vi "SwerveAssistHeading.vi"(1 "Joystick X":dbl, 2 "Joystick Y":dbl, 3 "In Deadband":bool, 4 "Joystick Rotation":dbl, 5 "Rotation Maximum":dbl=1.0, 6 "Locked Heading (deg) [0,360]":dbl format="%#_13g", 7 "Heading Angle PID":T1={"Kp"=0.1, "Ki"=0.1, "Kd"=0.1, "N-Diff"=10, "N-Int"=20, "Int Error Window"=0.5, "Max Ouput"=1.0, "Min Output"=-1.0, "Square Derivative"=FALSE, "N-Prop"=1} {"N-Prop" min=1; "Int Error Window" min=0.0; "N-Int" min=2; "N-Diff" min=2; "Kd" min=0.0; "Ki" min=0.0; "Kp" min=0.0}, 9 "Anti-Drift PID":T1={"Kp"=0.1, "Ki"=0.1, "Kd"=0.1, "N-Diff"=10, "N-Int"=20, "Int Error Window"=0.5, "Max Ouput"=1.0, "Min Output"=-1.0, "Square Derivative"=FALSE, "N-Prop"=1} {"N-Prop" min=1; "Int Error Window" min=0.0; "N-Int" min=2; "N-Diff" min=2; "Kd" min=0.0; "Ki" min=0.0; "Kp" min=0.0}, 10 "Orientation Mode":enum16{"Robot-Oriented", "Field-Oriented"}(ring), 11 "Heading Fudge Max (deg)":dbl=10.0, 13 "Deceleration Hysteresis (ms)":u32=250) -> (14 "Heading PID Plot":T2, 17 "In Deadband":bool, 18 "Assisted Rotation":dbl, 19 "Heading Assist On":bool)   [LabVIEW 2020]
doc: "This VI runs PID controllers to maintain the robot's heading using either (1) a locked heading angle or (2) preventing the robot from drifting while translating above a specified velocity. Dropping below the velocity threshold or manually commanding a rotation will switch off the anti-drift heading lock."
uses:
  b65aea0e-782f-4c6a-b3da-6b6dab4b3ae4.vi
  GlobalDrivebase.vi
  GlobalPoseAndTargeting.vi
  GlobalDriverStationData.vi
  GlobalDriverStationCommands.vi
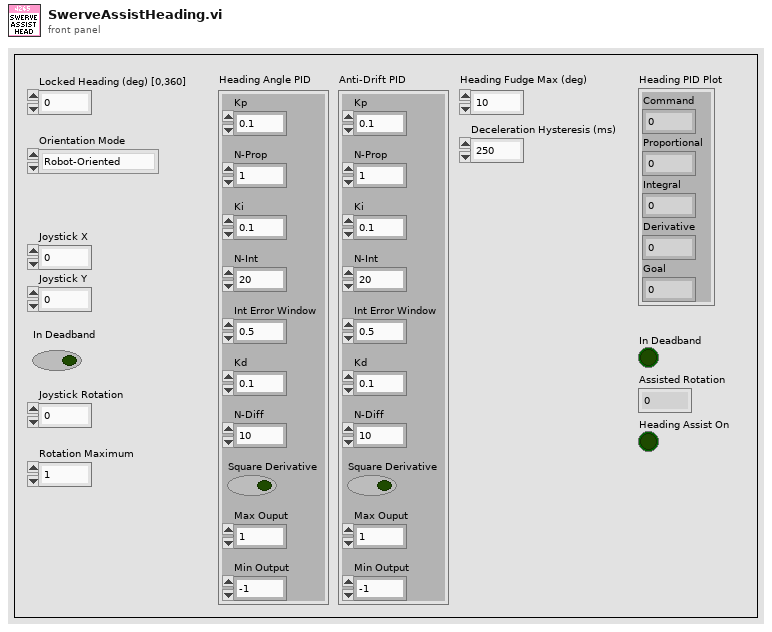
[diagram p1: front panel]
types:
  T1 = cluster{"Kp":dbl, "Ki":dbl, "Kd":dbl, "N-Diff":i32, "N-Int":i32, "Int Error Window":dbl, "Max Ouput":dbl, "Min Output":dbl, "Square Derivative":bool, "N-Prop":i32}
  T2 = cluster{"Command":dbl, "Proportional":dbl, "Integral":dbl, "Derivative":dbl, "Goal":dbl}
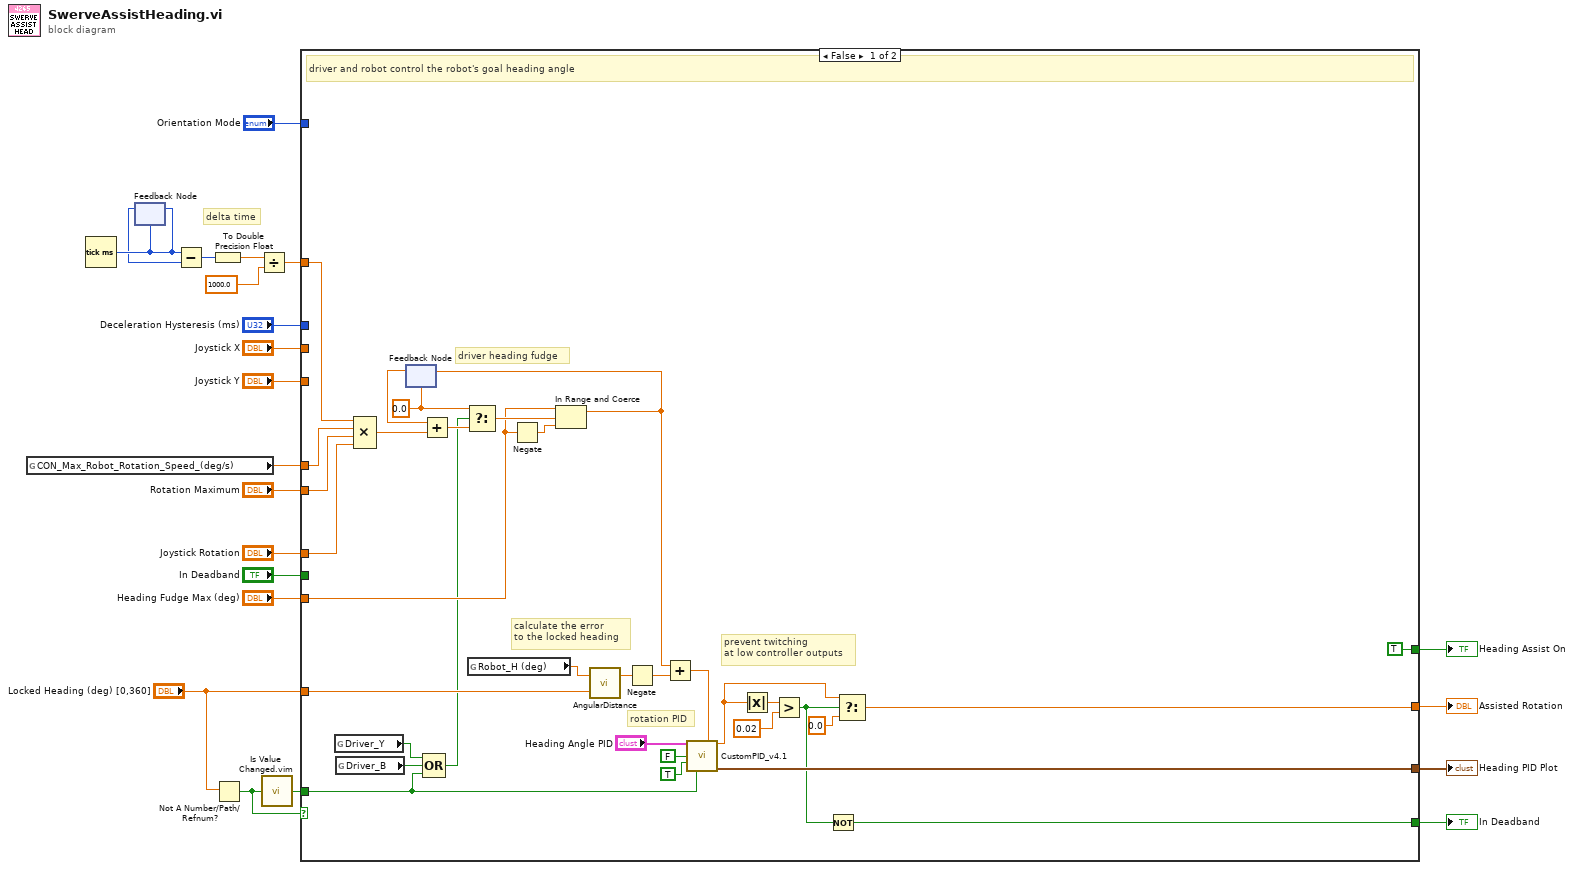
[diagram p0: block diagram]
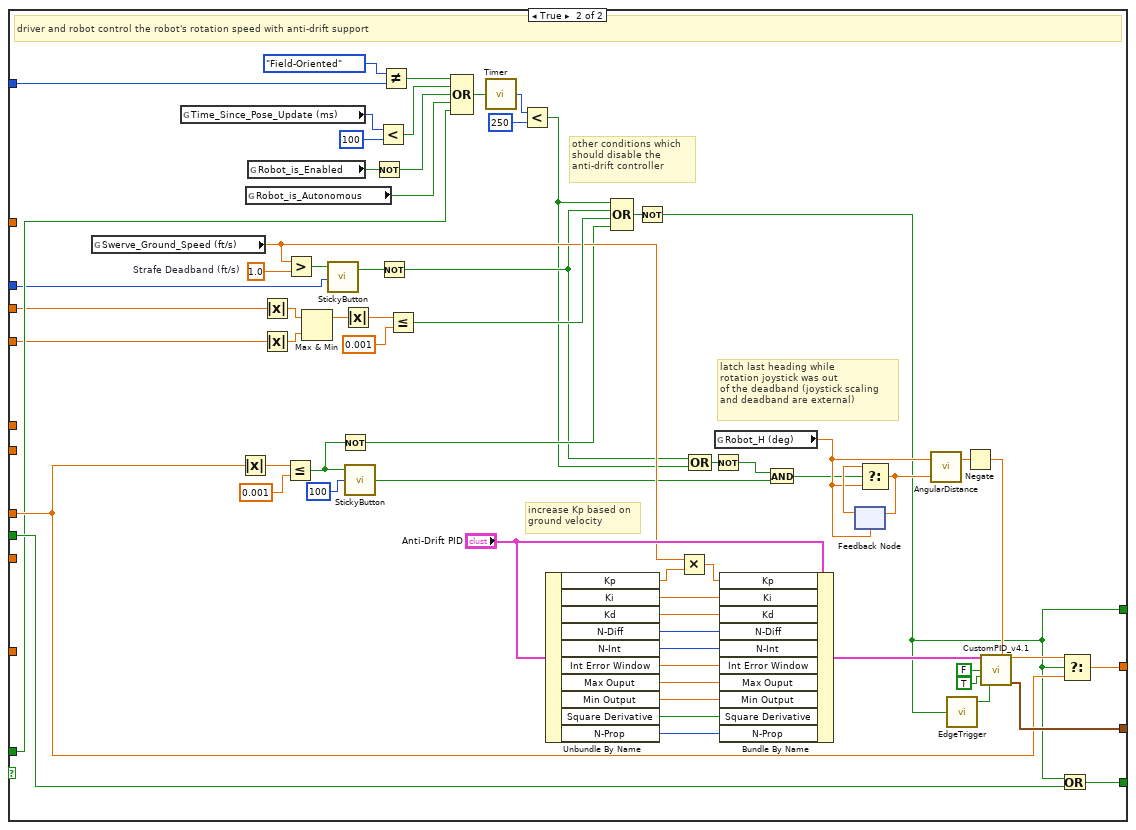
[diagram p2: hidden frame]
diagram:
  # "delta time"
  n1 = global read "GlobalDrivebase.vi" "CON_Max_Robot_Rotation_Speed_(deg/s)"() -> (w17:dbl)
  n2 = Tick Count (ms)() -> (millisecond timer value=w16:u32)
  n3 = feedback #1(w16) -> (w15:u32)
  n4 = feedback-in #1(w16) -> ()
  n5 = Subtract(x=w16, y=w15) -> (x-y=w14:u32)
  n6 = To Double Precision Float(number=w14) -> (double precision float=w13:dbl)
  n7 = Not A Number/Path/Refnum?(number/path/refnum="Locked Heading (deg) [0,360]") -> (NaN/Path/Refnum?=w20:bool)
  n8 = Divide(x=w13, y=1000.0) -> (x/y=w11:dbl)
  n9 = call "Is Value Changed.vim"("value"=w20) -> ("changed or first call?"=w5:bool)
  n10 = case shown="False" w20 {
    tunnel: "Locked Heading (deg) [0,360]" -> [w48 _]
    tunnel: [w47 w83] -> w8
    tunnel: "Joystick Rotation" -> [w38 w81]
    tunnel: [w42 w82] -> w9
    tunnel: [w28 w80] -> w7
    tunnel: w5 -> [w25 w63]
    tunnel: "In Deadband" -> [_ w79]
    tunnel: w17 -> [w40 _]
    tunnel: "Rotation Maximum" -> [w39 _]
    tunnel: w11 -> [w37 _]
    tunnel: "Heading Fudge Max (deg)" -> [w30 _]
    tunnel: [TRUE w78] -> w6
    tunnel: "Deceleration Hysteresis (ms)" -> [_ w62]
    tunnel: "Joystick Y" -> [_ w58]
    tunnel: "Joystick X" -> [_ w57]
    tunnel: "Orientation Mode" -> [_ w56]
    frame False {
      w33 = 0.0
      # "driver heading fudge"
      # "prevent twitching\nat low controller outputs"
      # "rotation PID"
      # "calculate the error\nto the locked heading"
      # "driver and robot control the robot's goal heading angle"
      n11 = global read "GlobalDriverStationCommands.vi" "Driver_Y"() -> (w23:bool)
      n12 = global read "GlobalDriverStationCommands.vi" "Driver_B"() -> (w26:bool)
      n13 = Compound Arithmetic op=MULTIPLY(w37, w40, w39, w38) -> (w36:dbl)
      n14 = feedback #2(w33) -> (w34:dbl)
      n15 = Add(x=w34, y=w36) -> (x+y=w35:dbl)
      n16 = Compound Arithmetic op=OR(w23, w26, w25) -> (w24:bool)
      n17 = Select(t=w33, s=w24, f=w35) -> (s? t:f=w31:dbl)
      n18 = global read "GlobalPoseAndTargeting.vi" "Robot_H (deg)"() -> (w55:dbl)
      n19 = Negate(x=w30) -> (-x=w32:dbl)
      n20 = In Range and Coerce(upper limit=w30, x=w31, lower limit=w32) -> (coerced(x)=w29:dbl)  [unwired: 1 out]
      n21 = feedback-in #2(w29) -> ()
      n22 = call "AngularDistance.vi"("Goal Angle (deg) [0,360]"=w48, "Current Angle (deg) [-Inf,+Inf]"=w55) -> ("Signed Angular Distance (deg) [-180,+180]"=w54:dbl)  [unwired: 1 out]
      n23 = Negate(x=w54) -> (-x=w49:dbl)
      n24 = Add(x=w29, y=w49) -> (x+y=w53:dbl)
      n25 = call "CustomPID_v4.1.vi"("PID Tuning Parameters"="Heading Angle PID", "Custom Error Calculation"=w53, "Reset on Goal Change ?"=FALSE, "Use Custom Error Calculation ?"=TRUE, "Reinit"=w25) -> ("Command"=w44:dbl, "Controller Summary"=w47:T2)  [unwired: 7 in, 2 out]
      n26 = Absolute Value(x=w44) -> (abs(x)=w46:dbl)
      n27 = Greater?(x=w46, y=0.02) -> (0:w41:bool)
      n28 = Not(x=w41) -> (.not. x?=w28:bool)
      n29 = Select(t=w44, s=w41, f=0.0 ("t")) -> (s? t:f=w42:dbl)
    }
    frame True {
      w112 = 1.0  # Strafe Deadband (ft/s)
      # "other conditions which\nshould disable the\nanti-drift controller"
      # "increase Kp based on\nground velocity"
      # "latch last heading while\nrotation joystick was out \nof the deadband (joystick scaling \nand deadband are external)"
      # "driver and robot control the robot's rotation speed with anti-drift support"
      n30 = global read "GlobalPoseAndTargeting.vi" "Swerve_Ground_Speed (ft/s)"() -> (w93:dbl)
      n31 = global read "GlobalPoseAndTargeting.vi" "Time_Since_Pose_Update (ms)"() -> (w70:u32)
      n32 = Absolute Value(x=w81) -> (abs(x)=w117:dbl)
      n33 = global read "GlobalDriverStationData.vi" "Robot_is_Autonomous"() -> (w67:bool)
      n34 = global read "GlobalDriverStationData.vi" "Robot_is_Enabled"() -> (w69:bool)
      n35 = Absolute Value(x=w57) -> (abs(x)=w61:dbl)
      n36 = Absolute Value(x=w58) -> (abs(x)=w60:dbl)
      n37 = Less Or Equal?(x=w117, y=0.001) -> (x <= y?=w85:bool)
      n38 = Greater?(x=w93, y=w112) -> (0:w87:bool)
      n39 = Max & Min(x=w61, y=w60) -> (max(x,y)=w59:dbl)  [unwired: 1 out]
      n40 = call "StickyButton.vi"("Time threshold (ms)"=w62, "Button Input"=w87) -> ("Sticky Button"=w88:bool)  [unwired: 1 in]
      n41 = Not(x=w85) -> (.not. x?=w66:bool)
      n42 = Absolute Value(x=w59) -> (abs(x)=w98:dbl)
      n43 = call "StickyButton.vi"("Time threshold (ms)"=u32 100 ("y"), "Button Input"=w85) -> ("Sticky Button"=w86:bool)  [unwired: 1 in]
      n44 = Not(x=w69) -> (.not. x?=w68:bool)
      n45 = Less?(x=w70, y=u32 100) -> (x < y?=w76:bool)
      n46 = Not(x=w88) -> (.not. x?=w65:bool)
      n47 = Not Equal?(x=enum16{"Robot-Oriented", "Field-Oriented"}."Field-Oriented", y=w56) -> (x != y?=w75:bool)
      n48 = Less Or Equal?(x=w98, y=0.001) -> (x <= y?=w96:bool)
      n49 = Compound Arithmetic op=OR(w75, w76, w68, w67, w63) -> (w73:bool)
      n50 = call "Timer.vi"("Reset Timer"=w73) -> ("Time (ms)"=w74:u32)
      n51 = Less?(x=w74, y=u32 250) -> (x < y?=w64:bool)
      n52 = Unbundle By Name("Anti-Drift PID") -> ("Kp"=w94:dbl, "Ki"=w89:dbl, "Kd"=w108:dbl, "N-Diff"=w107:i32, "N-Int"=w106:i32, "Int Error Window"=w105:dbl, "Max Ouput"=w104:dbl, "Min Output"=w103:dbl, "Square Derivative"=w102:bool, "N-Prop"=w101:i32)
      n53 = Compound Arithmetic op=OR(w64, w65, w96, w66) -> (w113:bool)
      n54 = Not(x=w113) -> (.not. x?=w78:bool)
      n55 = Multiply(x=w93, y=w94) -> (x*y=w92:dbl)
      n56 = Compound Arithmetic op=OR(w65, w64) -> (w95:bool)
      n57 = Not(x=w95) -> (.not. x?=w111:bool)
      n58 = global read "GlobalPoseAndTargeting.vi" "Robot_H (deg)"() -> (w114:dbl)
      n59 = Bundle By Name(cluster="Anti-Drift PID", "Kp"=w92, "Ki"=w89, "Kd"=w108, "N-Diff"=w107, "N-Int"=w106, "Int Error Window"=w105, "Max Ouput"=w104, "Min Output"=w103, "Square Derivative"=w102, "N-Prop"=w101) -> (w100:T1)
      n60 = And(x=w111, y=w86) -> (x .and. y?=w110:bool)
      n61 = feedback #3(w114) -> (w115:dbl)
      n62 = Select(t=w115, s=w110, f=w114) -> (s? t:f=w118:dbl)
      n63 = feedback-in #3(w118) -> ()
      n64 = call "AngularDistance.vi"("Goal Angle (deg) [0,360]"=w118, "Current Angle (deg) [-Inf,+Inf]"=w114) -> ("Signed Angular Distance (deg) [-180,+180]"=w91:dbl)  [unwired: 1 out]
      n65 = call "EdgeTrigger.vi"("Input Signal"=w78) -> ("Rising Edge Trigger"=w119:bool)  [unwired: 2 out]
      n66 = Negate(x=w91) -> (-x=w90:dbl)
      n67 = call "CustomPID_v4.1.vi"("PID Tuning Parameters"=w100, "Custom Error Calculation"=w90, "Reset on Goal Change ?"=FALSE, "Use Custom Error Calculation ?"=TRUE, "Reinit"=w119) -> ("Command"=w99:dbl, "Controller Summary"=w83:T2)  [unwired: 7 in, 2 out]
      n68 = Or(x=w78, y=w79) -> (x .or. y?=w80:bool)
      n69 = Select(t=w99, s=w78, f=w81) -> (s? t:f=w82:dbl)
    }
  }
  "Assisted Rotation" <- w9
  "Heading Assist On" <- w6
  "Heading PID Plot" <- w8
  "In Deadband" <- w7
